vi "Set ROI entry window UI from file-Boolean.vi"(8 "error in (no error)":errorcluster, 9 "Keys setup.Boolean":T2, 10 "Section name":string, 11 "Refnum in":T1) -> (0 "error out":errorcluster, 3 "Refnum out":T1)   [LabVIEW 2017]
uses:
  Typedefs/Ini file interface (Boolean).ctl
  <vilib>/Utility/config.llb/Config Data RefNum.ctl
  User Interface/ROI Entry screen/Globals/gl_ROI Entry UI globals.vi
  <vilib>/Utility/config.llb/NI_LVConfig.lvlib
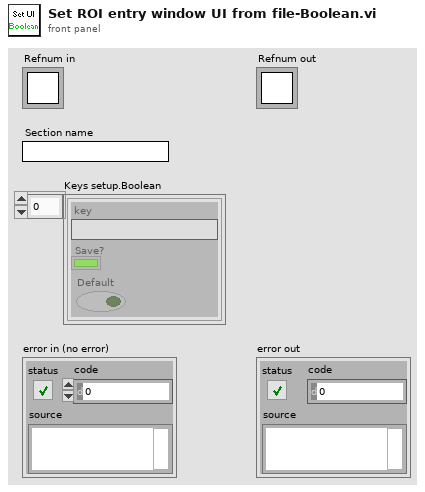
[diagram p1: front panel]
types:
  T1 = typedef "NI_LVConfig.lvlib/Config Data RefNum.ctl" = refnum<k1>
  T2 = typedef "Ini file interface (Boolean).ctl" = cluster{"key":string, "Save?":bool, "Default":bool}[]
  T3 = typedef "ROI entry screen ctrl refs cluster.ctl" = cluster{"Done button":refnum<vi>, "Imaging button":refnum<vi>, "Acquisition button":refnum<vi>, "POI dwell time (us)":refnum<vi>, "Scan dwell time per pixel (us)":refnum<vi>, "# of planes":refnum<vi>, "Zoom Ctrl":refnum<vi>, "Equal size":refnum<vi>, "Channel":refnum<vi>, "Image Display":refnum<vi>, "Z-Plane Selector":refnum<vi>, "Number of lines left":refnum<vi>, "Z-stack folder path":refnum<vi>, "POI Density":refnum<vi>, "Arb Plane Entry":refnum<vi>, "Whole plane":refnum<vi>, "Clear Last":refnum<vi>, "Clear All":refnum<vi>, "Trial Length (sec)":refnum<vi>, "Palette Type":refnum<vi>, "Intensity slider":refnum<vi>, "# POI":refnum<vi>, "Max Z Proj":refnum<vi>, "Zplane ind":refnum<vi>, "Wavelength (nm)":refnum<vi>, "Number of Trials":refnum<vi>, "Funct stim.trig.enable":refnum<vi>, "Funct stim.trig.delay (s)":refnum<vi>, "Line Mode":refnum<vi>, "Step size (µm)":refnum<vi>, "ROI move mode":refnum<vi>, "Cool-down time (s)":refnum<vi>, "Enable cool-down time":refnum<vi>, "Motor Z ind. (um)":refnum<vi>, "AOL Z ind. (um)":refnum<vi>, "Load Reference Image":refnum<vi>}
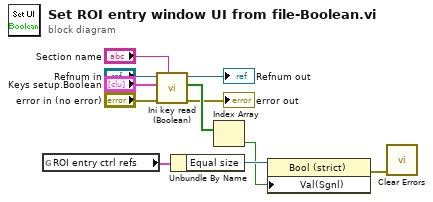
[diagram p0: block diagram]
diagram:
  n1 = global read "gl_ROI Entry UI globals.vi" "ROI entry ctrl refs"() -> (w2:T3)
  n2 = call "Ini key read (Boolean).vi"("Section"="Section name", "error in (no error)"="error in (no error)", "Parameter names & setup"="Keys setup.Boolean", "Ini file refnum in"="Refnum in") -> ("error out"=→"error out":errorcluster, "Value read/used"=w11:bool[], "Ini file refnum out"=→"Refnum out":T1)  [unwired: 5 in]
  n3 = Unbundle By Name(w2) -> ("Equal size"=w4:refnum<vi>)
  n4 = Index Array(array=w11) -> (element=w1:bool)  [unwired: 1 in]
  n5 = property class="Bool (strict)"(reference=w4, "Val(Sgnl)"=w1) -> (error out=w3:errorcluster)  [unwired: 1 in, 1 out]
  n6 = call <vilib>:"Clear Errors.vi"("error in (no error)"=w3) -> ()  [unwired: 5 in, 2 out]
